vi "Start Sync.vi"(8 "error in (no error)":errorcluster, 11 "gRPC Server in":refnum<class "GreeterService.lvclass">) -> (0 "error out":errorcluster, 3 "gRPC Server out":refnum<class "GreeterService.lvclass">)   [LabVIEW 2019, in "Generated_server.lvlib" / "GreeterService.lvclass"]
uses:
  GreeterService.lvclass
  GreeterService.lvclass/GreeterService.ctl
  RPC Messages/Greeter_req_req_oneof/Greeter_req_req_oneof.lvclass
  RPC Messages/Greeter_res_res_oneof/Greeter_res_res_oneof.lvclass
  RPC Messages/Greeter_res.ctl
  Generated_server.lvlib
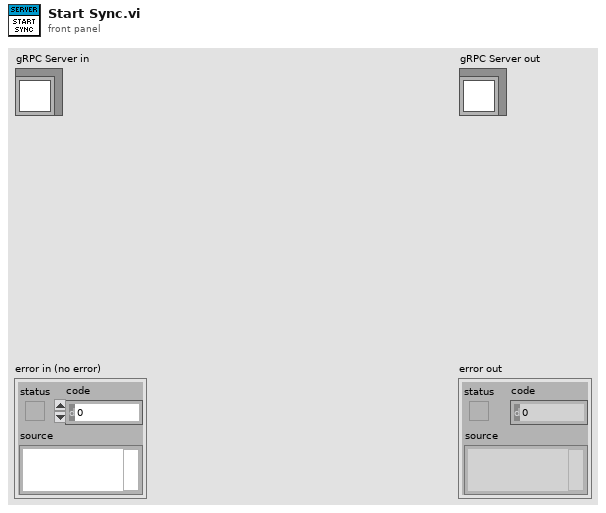
[diagram p1: front panel]
types:
  T1 = typedef "Generated_server.lvlib/Greeter_res.ctl" = cluster{"res_id":i32, "Greeter_res_res_oneof":refnum<class "Greeter_res_res_oneof.lvclass">}
  T2 = typedef "Generated_server.lvlib/GreeterService.lvclass/Server Internal UEs.ctl" = cluster{"GreeterService GetFeature Internal UE":refnum<user-event>}
  T3 = typedef "Generated_server.lvlib/GreeterService.lvclass/Server gRPC UEs.ctl" = cluster{"GreeterService GetFeature gRPC UE":refnum<user-event>}
  T4 = typedef "grpc-lvsupport-release.lvlib/grpcId.ctl" = u64
  T5 = typedef "Generated_server.lvlib/Greeter_req.ctl" = cluster{"req_id":i32, "Greeter_req_req_oneof":refnum<class "Greeter_req_req_oneof.lvclass">}
  T6 = typedef "grpc-lvsupport.lvlib/grpcId.ctl" = u64
  T7 = typedef "Generated_server.lvlib/Greeter_MessageA.ctl" = cluster{"data_a1":string}
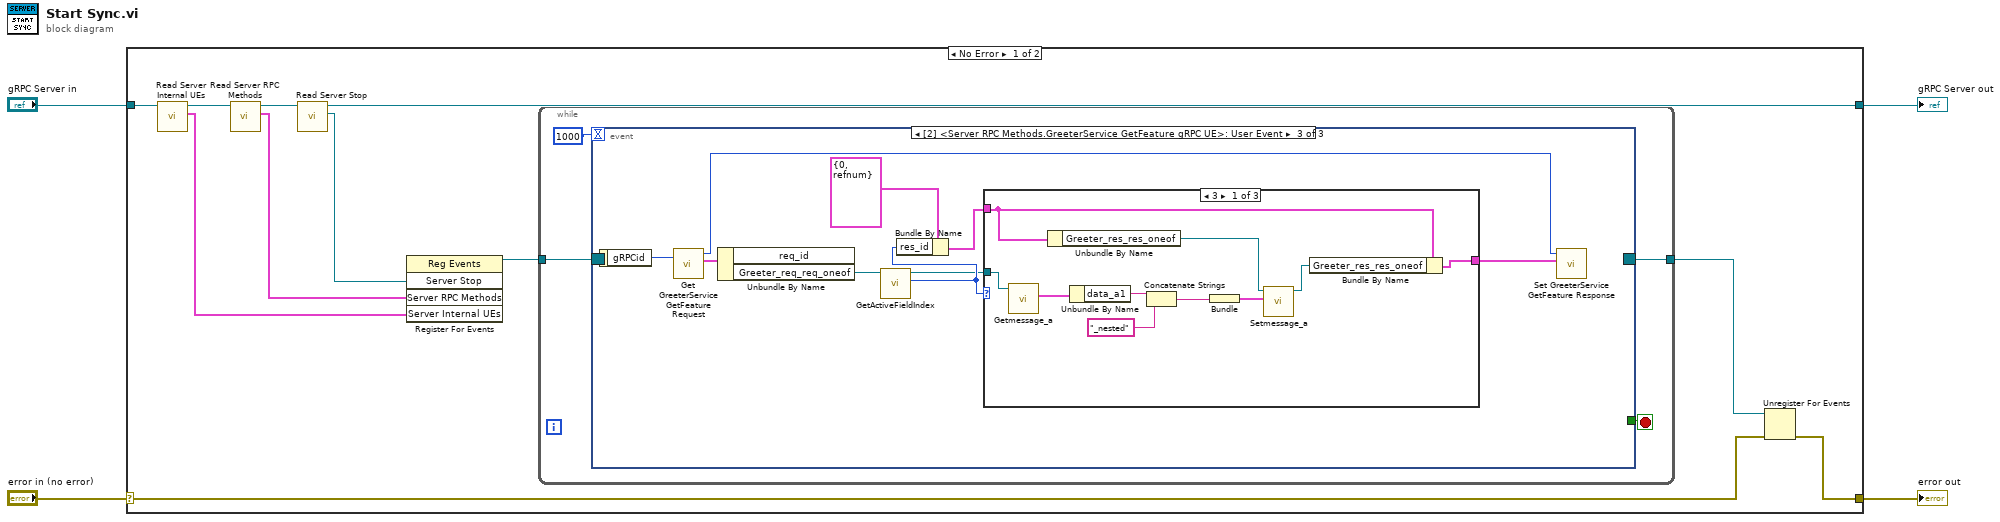
[diagram p0: block diagram]
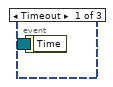
[diagram p2: hidden frame]
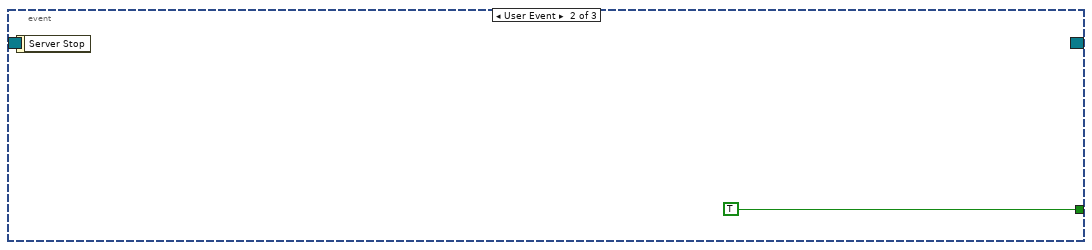
[diagram p3: hidden frame]
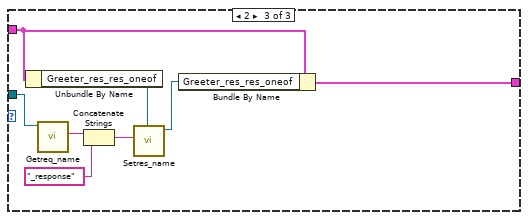
[diagram p5: hidden frame]
diagram:
  n1 = case shown="No Error" "error in (no error)" {
    selector: "error in (no error)" -> [w9 w50]
    tunnel: [w8 w50] -> w3
    tunnel: [w6 w49] -> w1
    tunnel: "gRPC Server in" -> [w15 w49]
    frame No Error {
      n2 = call "Read Server Internal UEs.vi"("SignalGeneratorService in"=w15) -> ("Server Internal UEs"=w13:T2, "SignalGeneratorService out"=w14:refnum<class "GreeterService.lvclass">)  [unwired: 8 in, 1 out]
      n3 = call "Read Server RPC Methods.vi"("SignalGeneratorService in"=w14) -> ("Server RPC Methods"=w7:T3, "SignalGeneratorService out"=w12:refnum<class "GreeterService.lvclass">)  [unwired: 8 in, 1 out]
      n4 = call-dynamic "Read Server Stop.vi"("iService in"=w12) -> ("Server Stop"=w5:refnum<user-event>, "iService out"=w6:refnum<class "GreeterService.lvclass">)  [unwired: 8 in, 1 out]
      n5 = register-events(w5, w7, w13) -> (reference out=w11:refnum<event-registration>)  [unwired: 2 in, 1 out]
      n6 = while {
        tunnel: w11 -> [w19]
        tunnel: [w17] -> w10
        stop <- w18 stop-if-true
        n7 = event "RPC Methods Event Structure" shown="[2] <Server RPC Methods.GreeterService GetFeature gRPC UE>: User Event" {
          selector: w19 -> [_ _ _]
          dyn-events: [_ _ _] -> w17
          timeout: 1000 -> [_ _ _]
          tunnel: [_ TRUE _] -> w18
          event Timeout {
            n8 = event-data() -> ()  [unwired: 1 in, 1 out]
          }
          event User Event {
            n9 = event-data() -> ()  [unwired: 1 in, 1 out]
          }
          event User Event {
            n10 = event-data() -> ("gRPCid"=w29:T4)  [unwired: 1 in]
            n11 = call "Get GreeterService GetFeature Request.vi"("gRPCid in"=w29) -> ("Message Data"=w28:T5, "gRPCid out"=w21:T6)  [unwired: 8 in, 1 out]
            n12 = Unbundle By Name(w28) -> ("Greeter_req_req_oneof"=w27:refnum<class "Greeter_req_req_oneof.lvclass">)  [unwired: 1 out]
            n13 = call "GetActiveFieldIndex.vi"("OneOfTemplate in"=w27) -> ("Active Field Index"=w26:i32, "OneOfTemplate out"=w24:refnum<class "Greeter_req_req_oneof.lvclass">)  [unwired: 8 in, 1 out]
            n14 = Bundle By Name(cluster=T1 {"res_id"=0, "Greeter_res_res_oneof"=refnum} ("Greeter_res"), "res_id"=w26) -> (w25:T1)
            n15 = case shown="3" w26 {
              tunnel: w25 -> [w32 w40 w44]
              tunnel: w24 -> [w39 _ w48]
              tunnel: [w30 w40 w41] -> w22
              frame 3 {
                n16 = call "Getmessage_a.vi"("OneOfTemplate in"=w39) -> ("Get_Val"=w38:T7)  [unwired: 8 in, 2 out]
                n17 = Unbundle By Name(w32) -> ("Greeter_res_res_oneof"=w33:refnum<class "Greeter_res_res_oneof.lvclass">)
                n18 = Unbundle By Name(w38) -> ("data_a1"=w37:string)
                n19 = Concatenate Strings(w37, "_nested" ("string")) -> (w35:string)
                n20 = Bundle(w35) -> (w34:cluster{string})  [unwired: 1 in]
                n21 = call "Setmessage_a.vi"("Set_Val"=w34, "OneOfTemplate in"=w33) -> ("OneOfTemplate out"=w31:refnum<class "Greeter_res_res_oneof.lvclass">)  [unwired: 8 in, 1 out]
                n22 = Bundle By Name(cluster=w32, "Greeter_res_res_oneof"=w31) -> (w30:T1)
              }
              frame 0, Default {
              }
              frame 2 {
                n23 = Unbundle By Name(w44) -> ("Greeter_res_res_oneof"=w43:refnum<class "Greeter_res_res_oneof.lvclass">)
                n24 = call "Getreq_name.vi"("OneOfTemplate in"=w48) -> ("Get_Val"=w47:string)  [unwired: 8 in, 2 out]
                n25 = Concatenate Strings(w47, "_response" ("string")) -> (w45:string)
                n26 = call "Setres_name.vi"("Set_Val"=w45, "OneOfTemplate in"=w43) -> ("OneOfTemplate out"=w42:refnum<class "Greeter_res_res_oneof.lvclass">)  [unwired: 8 in, 1 out]
                n27 = Bundle By Name(cluster=w44, "Greeter_res_res_oneof"=w42) -> (w41:T1)
              }
            }
            n28 = call "Set GreeterService GetFeature Response.vi"("Message Data"=w22, "gRPCid in"=w21) -> ()  [unwired: 9 in, 1 out]
          }
        }
      }
      n29 = Unregister For Events(event registration refnum=w10, error in=w9) -> (error out=w8:errorcluster)
    }
    frame Error {
    }
  }
  "error out" <- w3
  "gRPC Server out" <- w1
